vi "r_from_voltage_divider.vi"(1 "Measured Voltage":dbl, 2 "Supplied Voltage":dbl, 3 "Known Resistance (Ohm)":dbl) -> (0 "Measured Resistance (Ohm)":dbl)   [LabVIEW 2019]
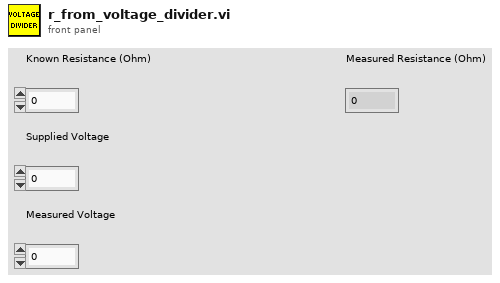
[diagram p1: front panel]
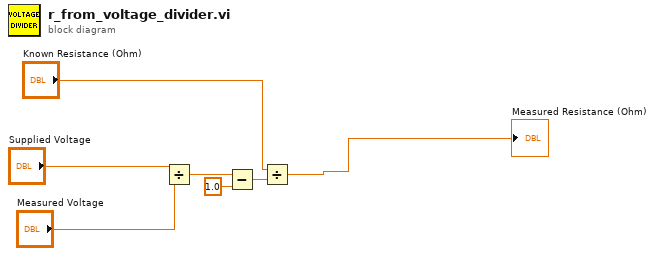
[diagram p0: block diagram]
diagram:
  n1 = Divide(x="Supplied Voltage", y="Measured Voltage") -> (x/y=w6:dbl)
  n2 = Subtract(x=w6, y=1.0) -> (x-y=w5:dbl)
  n3 = Divide(x="Known Resistance (Ohm)", y=w5) -> (x/y=→"Measured Resistance (Ohm)":dbl)
